vi "DataConversionFromBinaryFile.vi"(9 "file (use dialog)":path) -> (3 "Output Array":u32[](array[numeric]))   [LabVIEW 2015, in "VIPM2.lvlib"]
uses:
  VIPM2.lvlib
panel:
  out "Array":u32[](array[numeric])
  out "unsigned 32bit integer 2":u32 format="%x"
  out "x .or. y?":u32 format="%x"
  out "Numeric":i32
  out "size(Bytes)":i32
  out "NumberElementsArrayU32":u32
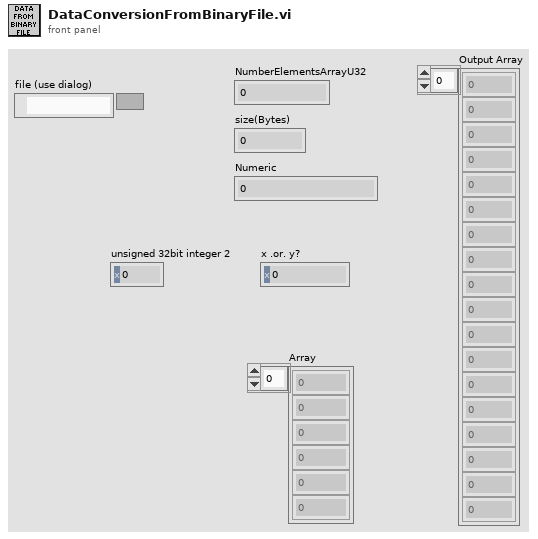
[diagram p1: front panel]
types:
  T1 = enum16{"big-endian, network order", "native, host order", "little-endian"}
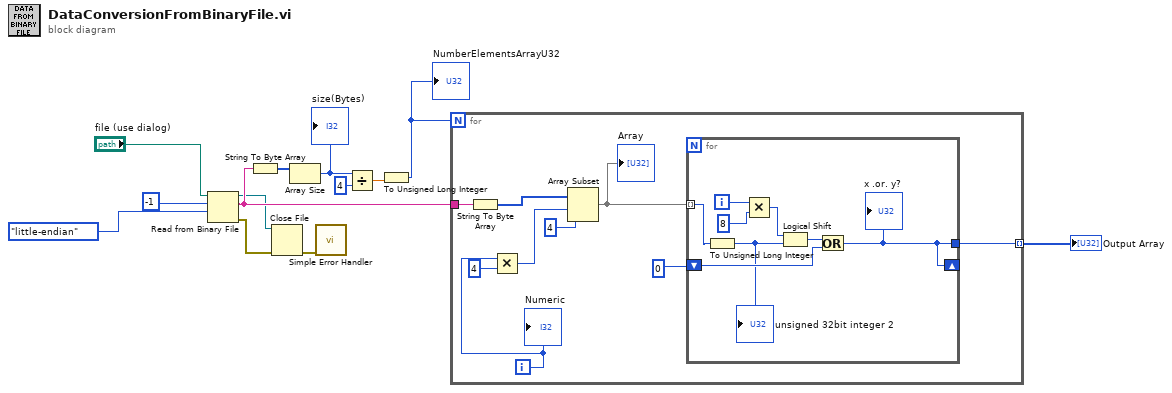
[diagram p0: block diagram]
diagram:
  n1 = Read from Binary File(9:T1."little-endian" ("byte order (0:big-endian, network order)"), 10:-1 ("count"), 11:"file (use dialog)") -> (0:w2:errorcluster, 2:w8:string, 3:w3:refnum<file>)  [unwired: 3 in, 1 out]
  n2 = String To Byte Array(string=w8) -> (unsigned byte array=w9:u8[])
  n3 = Close File(refnum=w3, error in=w2) -> (error out=w1:errorcluster)  [unwired: 1 out]
  n4 = Array Size(array=w9) -> (size(s)=w12:i32)
  "size(Bytes)" <- w12
  n5 = call <vilib>:"Simple Error Handler.vi"("error in (no error)"=w1) -> ()  [unwired: 4 in, 5 out]
  n6 = Divide(x=w12, y=4) -> (x/y=w11:dbl)
  n7 = To Unsigned Long Integer(number=w11) -> (unsigned 32bit integer=w10:u32)
  "NumberElementsArrayU32" <- w10
  n8 = for {
    N: w10 -> [_]
    tunnel: [w21] -> w4 mode=indexing
    tunnel: w8 -> [w19]
    i -> [w17]
    n9 = String To Byte Array(string=w19) -> (unsigned byte array=w18:u8[])
    n10 = Multiply(x=w17, y=4) -> (x*y=w15:i32)
    n11 = Array Subset(array=w18, index=w15, length=4) -> (w14:u8[])
    "Array" <- w14
    n12 = for {
      shift-right: [w25] -> _
      shift-left: 0 -> [w26]
      tunnel: [w25] -> w21
      tunnel: w14 -> [w23] mode=indexing
      i -> [w30]
      n13 = To Unsigned Long Integer(number=w23) -> (unsigned 32bit integer=w24:u32)
      "unsigned 32bit integer 2" <- w24
      n14 = Multiply(x=w30, y=8) -> (x*y=w28:i32)
      n15 = Logical Shift(y=w28, x=w24) -> (x << y=w27:u32)
      n16 = Or(x=w27, y=w26) -> (x .or. y?=w25:u32)
      "x .or. y?" <- w25
    }
    "Numeric" <- w17
  }
  "Output Array" <- w4
